vi "Iterate.vi"(8 "error in (no error)":errorcluster, 11 "Example Actor in":refnum<class "Example Actor.lvclass">) -> (0 "error out":errorcluster, 2 "Continue":bool, 3 "Example Actor out":refnum<class "Example Actor.lvclass">)   [LabVIEW 2021, in "Example Iterator NR Actor.lvlib" / "Example Actor.lvclass"]
doc: "Method called duriong the iterations"
uses:
  Example Actor.lvclass
  Example Actor.lvclass/Example Actor.ctl
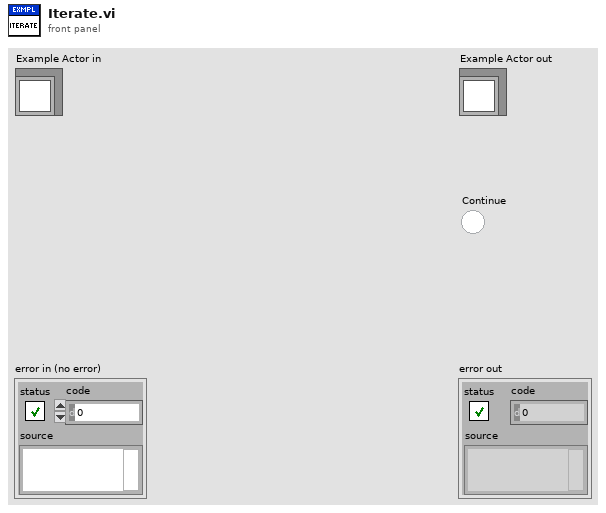
[diagram p1: front panel]
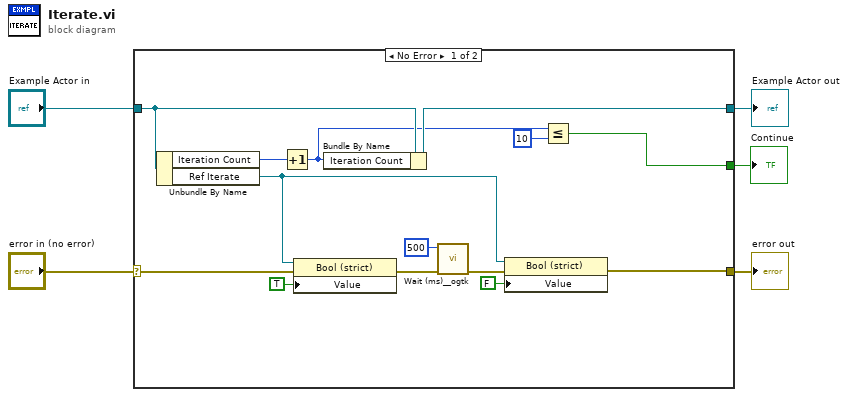
[diagram p0: block diagram]
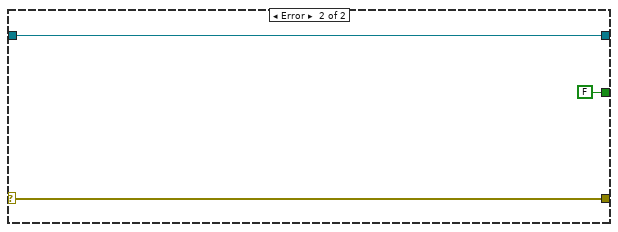
[diagram p2: hidden frame]
diagram:
  n1 = case shown="No Error" "error in (no error)" {
    selector: "error in (no error)" -> [w18 w22]
    tunnel: [w15 w22] -> w4
    tunnel: [w10 w21] -> w2
    tunnel: "Example Actor in" -> [w19 w21]
    tunnel: [w6 FALSE] -> w1
    frame No Error {
      n2 = Unbundle By Name(w19) -> ("Iteration Count"=w9:i32, "Ref Iterate"=w14:refnum<vi>)
      n3 = Increment(x=w9) -> (x+1=w8:i32)
      n4 = property class="Bool (strict)"(reference=w14, error in=w18, "Value"=TRUE) -> (error out=w17:errorcluster)  [unwired: 1 out]
      n5 = Bundle By Name(cluster=w19, "Iteration Count"=w8) -> (w10:refnum<class "Example Actor.lvclass">)
      n6 = call <userlib>:"Wait (ms)__ogtk.vi"("error in (no error)"=w17, "milliseconds to wait"=u32 500) -> ("error out"=w16:errorcluster)  [unwired: 8 in, 1 out]
      n7 = property class="Bool (strict)"(reference=w14, error in=w16, "Value"=FALSE) -> (error out=w15:errorcluster)  [unwired: 1 out]
      n8 = Less Or Equal?(x=w8, y=10) -> (x <= y?=w6:bool)
    }
    frame Error {
    }
  }
  "error out" <- w4
  "Example Actor out" <- w2
  "Continue" <- w1
